vi "Potentiometer PID (SubVI).vi"(4 "refnum name":string, 5 "Encoder Config":cluster{"Elevator Height":dbl, "Offset":dbl}, 6 "PID Settings":T1, 7 "PID Limits":cluster{"Upper Limit":dbl, "Lower Limit":dbl}) -> (3 "output":dbl)   [LabVIEW 2014]
uses:
  <vilib>/addons/control/pid/pid.llb/PID (DBL).vi
  <vilib>/addons/control/pid/NI_PID_pid.lvlib
panel:
  out "Potentiometer Distance Chart":dbl(graph)
  out "PID Output Chart":dbl(graph)
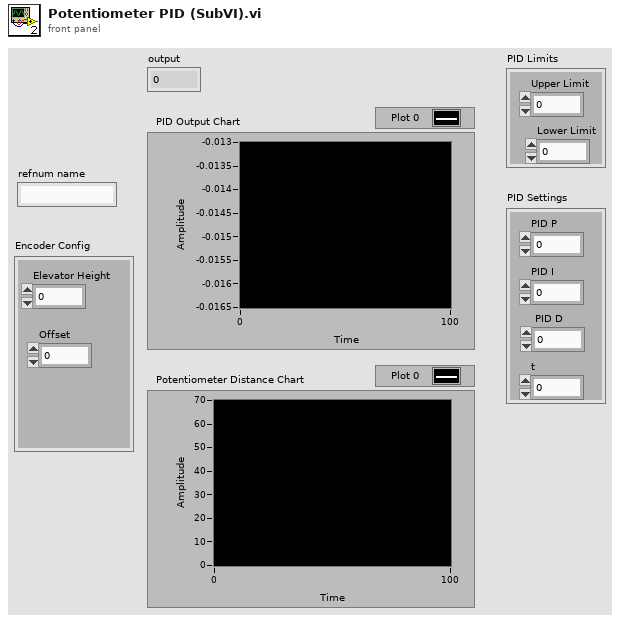
[diagram p1: front panel]
types:
  T1 = cluster{"PID P":dbl, "PID I":dbl, " PID D":dbl, "t":dbl}
  T2 = typedef "WPI_PotentiometerDevRef.ctl" = cluster{"DevStatus":errorcluster, "Controller":T3, "Analog Channel":T4, "Invert Output":bool}
  T3 = typedef "FPGA_TypedefAnalogModule.ctl" = enum16{"Controller 1"}
  T4 = typedef "FPGA_AIChannel.ctl" = enum8{"AI 0", "AI 1", "AI 2", "AI 3", "AI MXP 0", "AI MXP 1", "AI MXP 2", "AI MXP 3", "Invalid"}
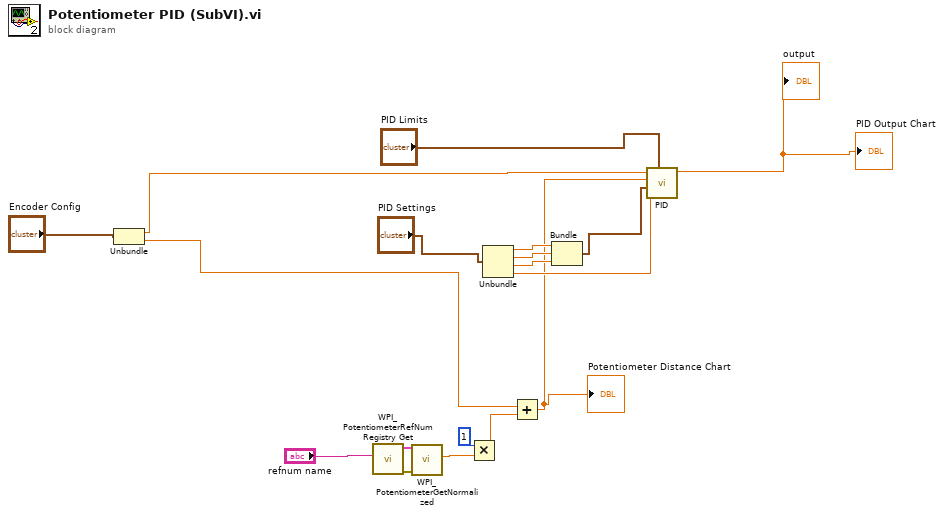
[diagram p0: block diagram]
diagram:
  n1 = Unbundle("Encoder Config") -> ("Elevator Height"=w2:dbl, "Offset"=w3:dbl)
  n2 = call <vilib>:"WPI_PotentiometerRefNum Registry Get.vi"("refnum name"="refnum name") -> ("error out"=w7:errorcluster, "PotDevRef"=w8:T2)  [unwired: 9 in]
  n3 = call <vilib>:"WPI_PotentiometerGetNormalized.vi"("error in"=w7, "PotDevRef"=w8) -> ("Normalized Value"=w6:dbl)  [unwired: 7 in, 2 out]
  n4 = Multiply(x=1, y=w6) -> (x*y=w4:dbl)
  n5 = Unbundle("PID Settings") -> ("PID P"=w15:dbl, "PID I"=w14:dbl, "PID D"=w13:dbl, "t"=w12:dbl)
  n6 = Add(x=w3, y=w4) -> (x+y=w10:dbl)
  "Potentiometer Distance Chart" <- w10
  n7 = Bundle("PID P"=w15, "PID I"=w14, "PID D"=w13) -> (w11:cluster{"PID P":dbl, "PID I":dbl, " PID D":dbl})  [unwired: 1 in]
  n8 = call-poly <vilib>:"PID.vi"("output range"="PID Limits", "dt (s)"=w12, "PID gains"=w11, "process variable"=w10, "setpoint"=w2) -> ("output"=→"PID Output Chart" →"output":dbl)  [unwired: 5 in, 1 out]
